vi "Car Wash Timer Kernel.vi"(7 "Proximity switch":bool, 8 "error in (no error)":errorcluster, 9 "Timer Data in":T1, 10 "Time Target (s)":dbl, 11 "Command":T3) -> (0 "error out":errorcluster, 1 "Timer Data out":T1, 3 "Status":T2)   [LabVIEW 2013]
doc: "This is the kernel of the car wash timer. The Timer Data cluster contains the state variables for the timer. Storage for the state variables should be provided in a shell VI."
uses:
  Type Defs/Car Wash Timer Enum.ctl
  Shared Files/Shared Type Defs/Cycle Status Cluster.ctl
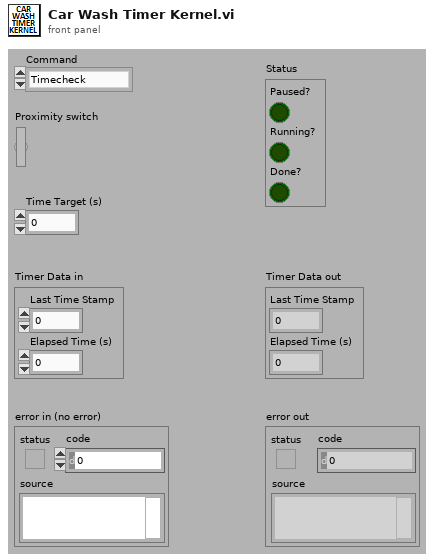
[diagram p1: front panel]
types:
  T1 = cluster{"Last Time Stamp":dbl, "Elapsed Time (s)":dbl}
  T2 = typedef "Cycle Status Cluster.ctl" = cluster{"Paused?":bool, "Running?":bool, "Done?":bool}
  T3 = typedef "Car Wash Timer Enum.ctl" = enum16{"Timecheck", "Reset"}
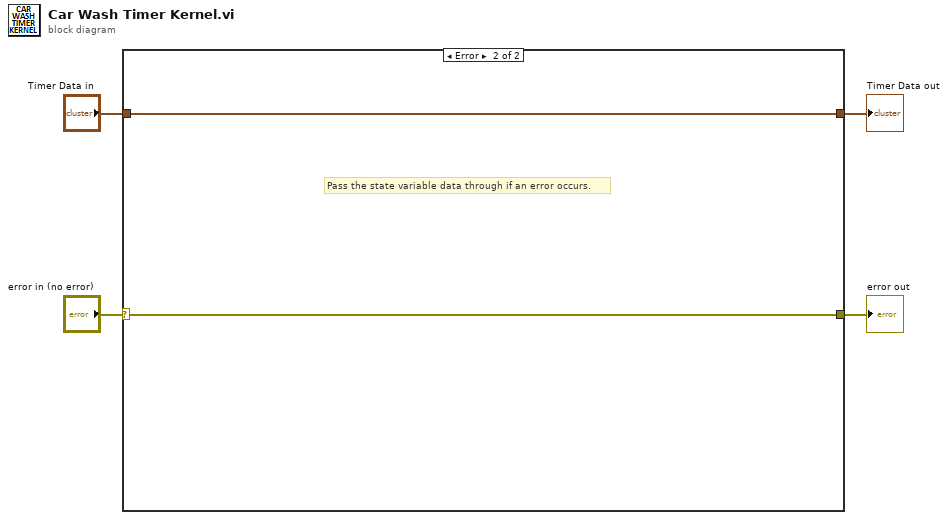
[diagram p0: block diagram]
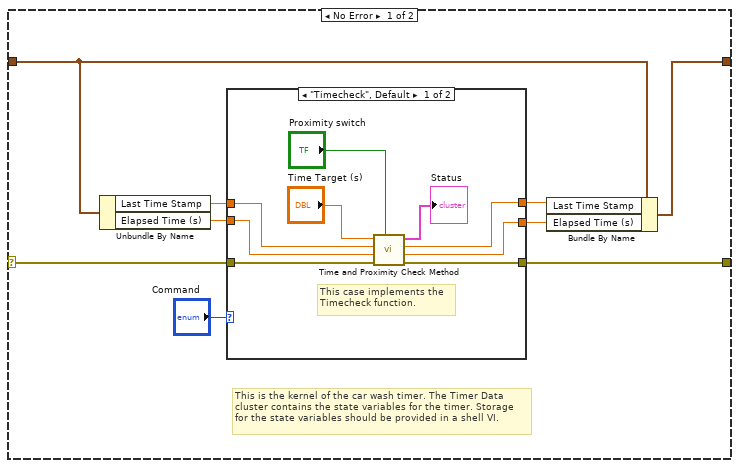
[diagram p2: hidden frame]
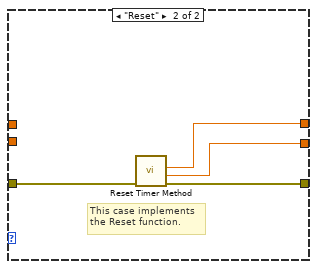
[diagram p3: hidden frame]
diagram:
  n1 = case shown="Error" "error in (no error)" {
    selector: "error in (no error)" -> [w8 w28]
    tunnel: [w7 w28] -> w3
    tunnel: "Timer Data in" -> [w6 w27]
    tunnel: [w5 w27] -> w1
    frame No Error {
      # "This is the kernel of the car wash timer. The Timer Data\ncluster contains the state variables for the timer. Storage\nfor the state variables should be provided in a shell VI."
      n2 = Unbundle By Name(w6) -> ("Last Time Stamp"=w12:dbl, "Elapsed Time (s)"=w11:dbl)
      n3 = case shown="\"Timecheck\", Default" "Command" {
        tunnel: w8 -> [w20 w26]
        tunnel: [w19 w25] -> w7
        tunnel: [w18 w23] -> w9
        tunnel: [w17 w24] -> w10
        tunnel: w12 -> [w15 _]
        tunnel: w11 -> [w14 _]
        frame "Timecheck", Default {
          # "This case implements the\nTimecheck function."
          n4 = call "Time and Proximity Check Method.vi"("Proximity switch"="Proximity switch", "error in (no error)"=w20, "Elapsed Time (s)"=w14, "Last Time Stamp"=w15, "Time Target (s)"="Time Target (s)") -> ("error out"=w19:errorcluster, "New Elapsed Time (s)"=w18:dbl, "New Time Stamp"=w17:dbl, "Status"=→"Status":T2)  [unwired: 3 in]
        }
        frame "Reset" {
          # "This case implements\nthe Reset function."
          n5 = call "Reset Timer Method.vi"("error in (no error)"=w26) -> ("error out"=w25:errorcluster, "New Elapsed Time (s)"=w23:dbl, "New Time Stamp"=w24:dbl)  [unwired: 8 in]
        }
      }
      n6 = Bundle By Name(cluster=w6, "Last Time Stamp"=w10, "Elapsed Time (s)"=w9) -> (w5:T1)
    }
    frame Error {
      # "Pass the state variable data through if an error occurs."
    }
  }
  "error out" <- w3
  "Timer Data out" <- w1
